vi "Get Axis Aligned Instructions.vi"(1 "Wall value":dbl, 2 "Key Points":i32[][](array[numeric]), 3 "obstacles":dbl[][](array[numeric])) -> (0 "AA Instructions":i32[][](array[numeric]))   [LabVIEW 2015]
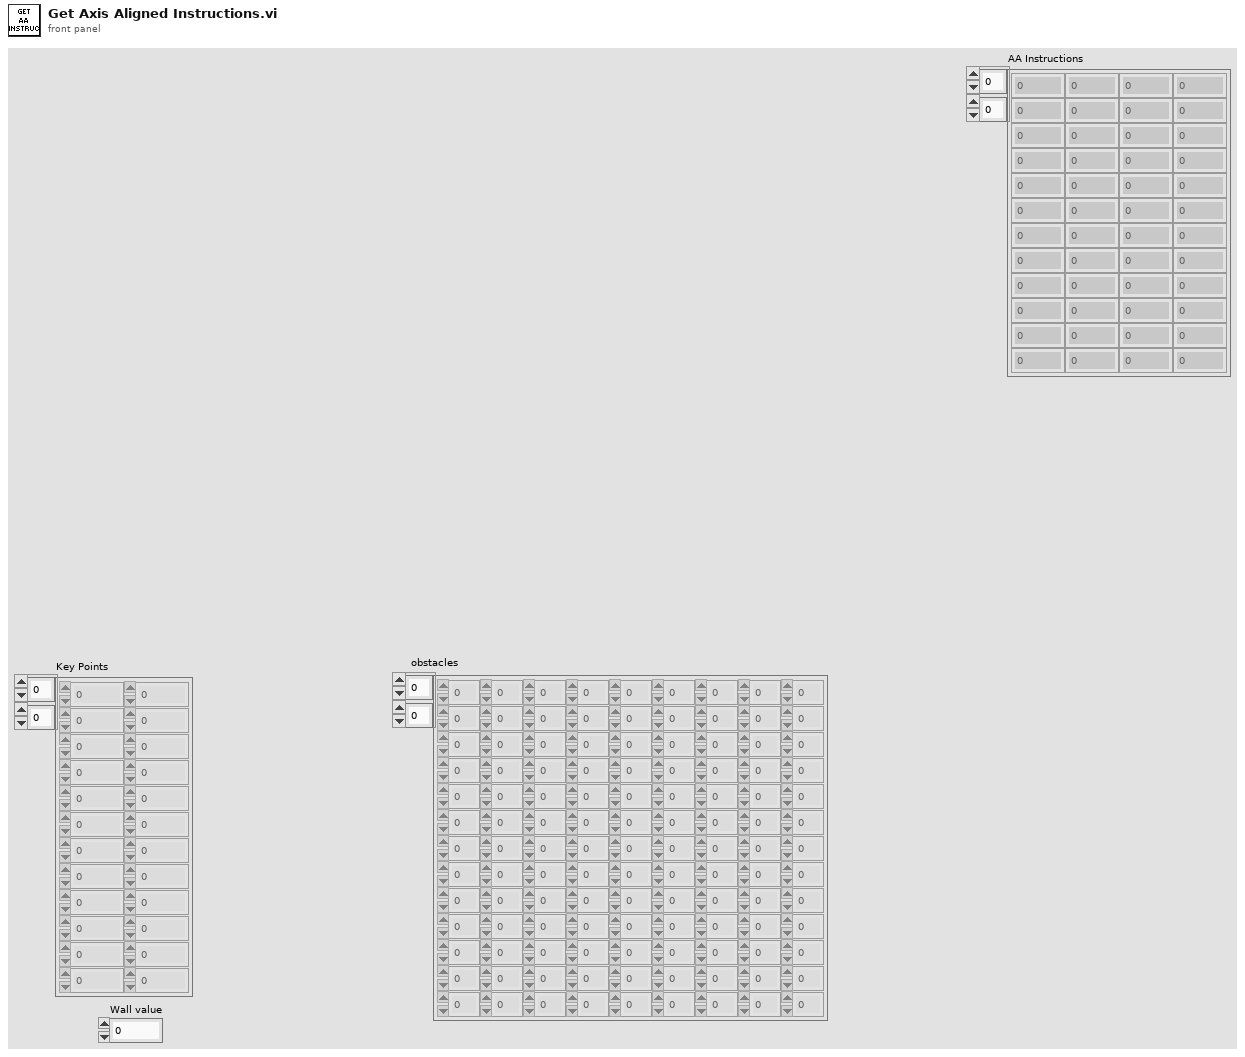
[diagram p1: front panel]
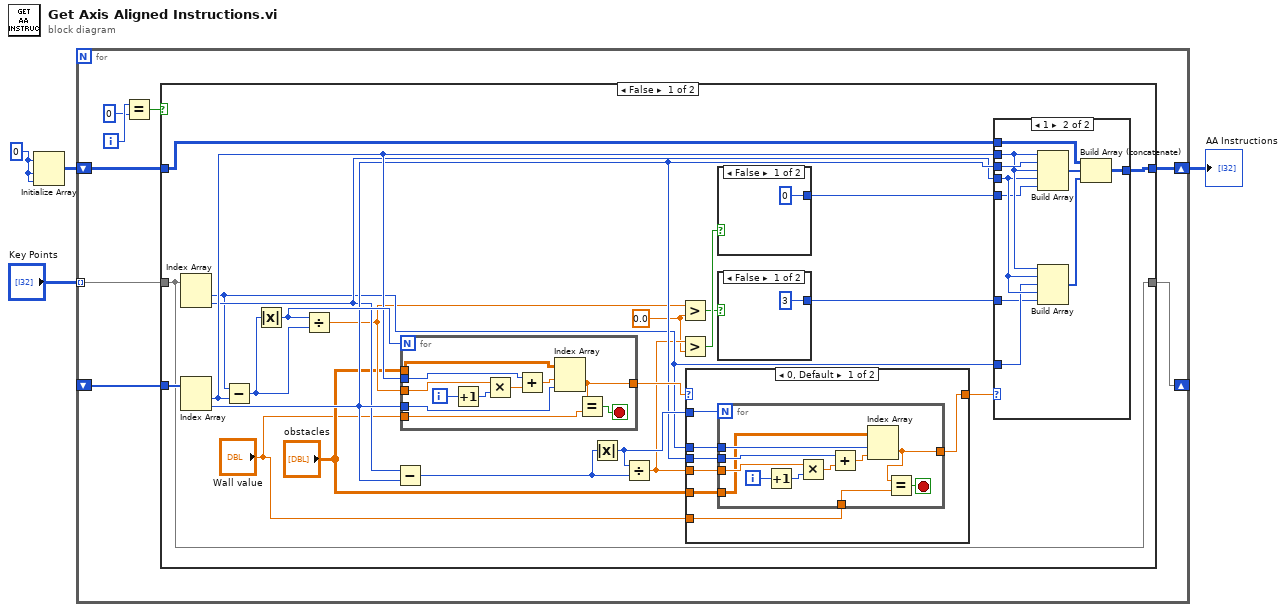
[diagram p0: block diagram]
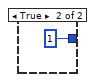
[diagram p2: hidden frame]
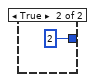
[diagram p3: hidden frame]
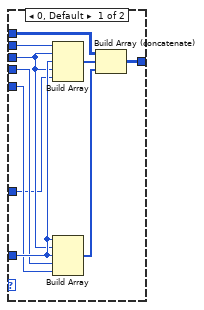
[diagram p4: hidden frame]
diagram:
  w3 = 0
  n1 = Initialize Array(w3, w3, w3) -> (w1:i32[][])
  n2 = for {
    shift-right: [w9] -> _
    shift-left: _ -> [w7]
    tunnel: "Key Points" -> [w8] mode=indexing
    shift-right: [w6] -> w2
    shift-left: w1 -> [w5]
    i -> [w12]
    n3 = Equal?(x=w12, y=0) -> (x = y?=w10:bool)
    n4 = case shown="False" w10 {
      tunnel: [w34 w91] -> w9
      tunnel: w8 -> [w34 w91]
      tunnel: w7 -> [w35 _]
      tunnel: w5 -> [w27 w90]
      tunnel: [w22 w90] -> w6
      frame False {
        w16 = 0.0 ("y")
        n5 = Index Array(array=w34) -> (element #1=w23:i32, element #2=w24:i32)  [unwired: 2 in]
        n6 = Index Array(array=w35) -> (element #1=w26:i32, element #2=w25:i32)  [unwired: 2 in]
        n7 = Subtract(x=w23, y=w26) -> (x-y=w33:i32)
        n8 = Absolute Value(x=w33) -> (abs(x)=w31:i32)
        n9 = Divide(x=w31, y=w33) -> (x/y=w17:dbl)
        n10 = Subtract(x=w24, y=w25) -> (x-y=w32:i32)
        n11 = for {
          N: w31 -> [_]
          tunnel: w17 -> [w87]
          tunnel: w26 -> [w85]
          tunnel: w25 -> [w83]
          tunnel: [w80] -> w30
          tunnel: "obstacles" -> [w82]
          tunnel: "Wall value" -> [w79]
          i -> [w89]
          stop <- w81 stop-if-true
          n12 = Increment(x=w89) -> (x+1=w88:i32)
          n13 = Multiply(x=w87, y=w88) -> (x*y=w86:dbl)
          n14 = Add(x=w85, y=w86) -> (x+y=w84:dbl)
          n15 = Index Array(array=w82, index (row)=w84, index (col)=w83) -> (element=w80:dbl)
          n16 = Equal?(x=w80, y=w79) -> (x = y?=w81:bool)
        }
        n17 = Absolute Value(x=w32) -> (abs(x)=w29:i32)
        n18 = Divide(x=w29, y=w32) -> (x/y=w21:dbl)
        n19 = Greater?(x=w17, y=w16) -> (0:w18:bool)
        n20 = Greater?(x=w21, y=w16) -> (0:w20:bool)
        n21 = case shown="0, Default" w30 {
          selector: w30 -> [_ w78]
          tunnel: w29 -> [w66 _]
          tunnel: w21 -> [w65 _]
          tunnel: w23 -> [w64 _]
          tunnel: w25 -> [w63 _]
          tunnel: [w62 w78] -> w28
          tunnel: "obstacles" -> [w61 _]
          tunnel: "Wall value" -> [w60 _]
          frame 0, Default {
            n22 = for {
              N: w66 -> [_]
              tunnel: w65 -> [w75]
              tunnel: w64 -> [w74]
              tunnel: w63 -> [w72]
              tunnel: [w69] -> w62
              tunnel: w61 -> [w70]
              tunnel: w60 -> [w68]
              i -> [w77]
              stop <- w67 stop-if-true
              n23 = Increment(x=w77) -> (x+1=w76:i32)
              n24 = Multiply(x=w75, y=w76) -> (x*y=w73:dbl)
              n25 = Add(x=w72, y=w73) -> (x+y=w71:dbl)
              n26 = Index Array(array=w70, index (row)=w74, index (col)=w71) -> (element=w69:dbl)
              n27 = Equal?(x=w69, y=w68) -> (x = y?=w67:bool)
            }
          }
          frame 1 {
          }
        }
        n28 = case shown="False" w20 {
          tunnel: [0 2] -> w19
          frame False {
          }
          frame True {
          }
        }
        n29 = case shown="False" w18 {
          tunnel: [3 1] -> w15
          frame False {
          }
          frame True {
          }
        }
        n30 = case shown="1" w28 {
          tunnel: w27 -> [w49 w59]
          tunnel: w26 -> [w48 w56]
          tunnel: w25 -> [w42 w58]
          tunnel: w24 -> [w45 w55]
          tunnel: w23 -> [w46 w54]
          tunnel: [w43 w52] -> w22
          tunnel: w19 -> [w41 w51]
          tunnel: w15 -> [w40 w50]
          frame 0, Default {
            n31 = Build Array(w48, w42, w46, w42, w40) -> (w47:i32[])
            n32 = Build Array(w46, w42, w46, w45, w41) -> (w44:i32[])
            n33 = Build Array (concatenate)(w49, w47, w44) -> (w43:i32[][])
          }
          frame 1 {
            n34 = Build Array(w56, w58, w56, w55, w51) -> (w57:i32[])
            n35 = Build Array(w56, w55, w54, w55, w50) -> (w53:i32[])
            n36 = Build Array (concatenate)(w59, w57, w53) -> (w52:i32[][])
          }
        }
      }
      frame True {
      }
    }
  }
  "AA Instructions" <- w2
